vi "TKEEP Array (True).vi"() -> (3 "tkeep":bool[](array[boolean]))   [LabVIEW 2023, in "CHDR Support.lvlib"]
doc: "Constant 32-bit TKeep (byte enable) array for a 256-bit word."
uses:
  CHDR Support.lvlib
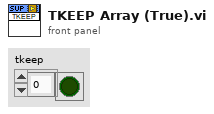
[diagram p1: front panel]
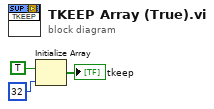
[diagram p0: block diagram]
diagram:
  n1 = Initialize Array(TRUE, 32 ("dimension size")) -> (→"tkeep":bool[])
